vi "Main.vi"() -> ()   [LabVIEW 2016]
doc: "The myRIO Project template acquires acceleration data from the onboard accelerometer and displays the changes of acceleration values in a waveform chart."
uses:
  <vilib>/myRIO/Instrument Drivers/Onboard IO/PWM/typedefs/PWM Reference.ctl
  <vilib>/myRIO/Common/Instrument Driver Framework/Utilities/typedefs/myRIO Generic Hardware Reference.ctl
  <vilib>/myRIO/Common/Instrument Driver Framework/Utilities/typedefs/Hardware Version Enum.ctl
  <vilib>/myRIO/Common/Instrument Driver Framework/Utilities/typedefs/myRIO v1.0 Reference.ctl
  <vilib>/myRIO/Common/Instrument Driver Framework/Utilities/typedefs/Generic FPGA Reference.ctl
  <vilib>/myRIO/Common/Instrument Driver Framework/myRIO v1.0/PWM/typedefs/PWM Channels Enum.ctl
  <vilib>/myRIO/Instrument Drivers/Onboard IO/PWM/typedefs/PWM Configuration.ctl
  <vilib>/userdefined/High Color/nirio_resource_hc.ctl
  <vilib>/myRIO/Common/Instrument Driver Framework/myRIO v1.0/PWM/vis/myRIO v1.1 Open PWM.vi
  <vilib>/myRIO/Common/Instrument Driver Framework/Utilities/vis/Validate Channels.vi
  <vilib>/myRIO/Common/Instrument Driver Framework/myRIO v1.0/PWM/vis/myRIO v1.0 Reserve PWM.vi
  <vilib>/myRIO/Instrument Drivers/Onboard IO/PWM/vis/Set Duty Cycle and Frequency.vi
  <vilib>/myRIO/Common/Instrument Driver Framework/myRIO v1.0/PWM/vis/myRIO v1.0 Close PWM.vi
  <vilib>/myRIO/Common/Instrument Driver Framework/myRIO v1.0/UART/vis/myRIO v1.0 Close UART.vi
  <vilib>/myRIO/Common/Instrument Driver Framework/myRIO v1.0/PWM/vis/myRIO v1.0 Build MUX Configuration PWM.vi
  <vilib>/myRIO/Common/Instrument Driver Framework/myRIO v1.0/Resource Manager/vis/myRIO v1.0 Reserve Channel List.vi
  <vilib>/myRIO/Common/Instrument Driver Framework/myRIO v1.0/PWM/vis/myRIO v1.0 Unreserve PWM.vi
  <vilib>/myRIO/Common/Instrument Driver Framework/myRIO v1.0/Resource Manager/vis/myRIO v1.0 Create Configuration List.vi
  <vilib>/myRIO/Common/Instrument Driver Framework/myRIO v1.0/Resource Manager/vis/myRIO v1.0 Reserve Channel.vi
  <vilib>/myRIO/Common/Instrument Driver Framework/myRIO v1.0/Resource Manager/vis/myRIO v1.0 Unreserve Channel.vi
  <vilib>/myRIO/Common/Instrument Driver Framework/myRIO v1.0/Resource Manager/vis/myRIO v1.0 Unreserve Channel List.vi
  <vilib>/myRIO/Common/Instrument Driver Framework/myRIO v1.0/Resource Manager/vis/myRIO v1.0 Build Mutex Name.vi
  <vilib>/Utility/VariantDataType/GetNumericInfo.vi
  <vilib>/Utility/error.llb/Error Cluster From Error Code.vi
  <vilib>/myRIO/Common/Instrument Driver Framework/myRIO v1.0/myRIO v1.1 Open.vi
  <vilib>/myRIO/Common/Instrument Driver Framework/Utilities/vis/IO Manager.vi
  <vilib>/myRIO/Common/Instrument Driver Framework/Utilities/vis/Configuration Manager.vi
  <vilib>/myRIO/Common/Instrument Driver Framework/myRIO v1.0/Resource Manager/vis/myRIO v1.0 Configure IO.vi
  <vilib>/myRIO/Common/Instrument Driver Framework/myRIO v1.0/myRIO v1.0 Close.vi
  <vilib>/myRIO/Common/Instrument Driver Framework/myRIO v1.0/PWM/vis/myRIO v1.0 Write PWM.vi
  <vilib>/myRIO/Common/Instrument Driver Framework/myRIO v1.0/PWM/vis/myRIO v1.0 Shutdown PWM.vi
  <vilib>/myRIO/Common/Instrument Driver Framework/Utilities/vis/FPGA Ref Manager.vi
  <vilib>/myRIO/Common/Instrument Driver Framework/myRIO v1.0/myRIO v1.0 Reset FPGA.vi
  <vilib>/myRIO/Common/Instrument Driver Framework/myRIO v1.0/IRQ/vis/myRIO v1.0 IRQ Info FGV.vi
  <vilib>/myRIO/Common/Instrument Driver Framework/myRIO v1.0/IRQ/vis/myRIO v1.0 Timer IRQ Info FGV.vi
  <vilib>/myRIO/Common/Instrument Driver Framework/myRIO v1.0/IRQ/vis/myRIO v1.0 ISR Agent.vi
  <vilib>/myRIO/Instrument Drivers/Onboard IO/PWM/vis/myRIO PWM Open.xnode
  <vilib>/myRIO/Instrument Drivers/Utilities/Utilities.lvlib
  <vilib>/myRIO/Instrument Drivers/Onboard IO/PWM/PWM.lvlib
panel:
  in  "Blue Duty Cycle":dbl(slide)=10.0 scale=0.0..10.0
  in  "Green Duty Cycle":dbl(slide)=10.0 scale=0.0..10.0
  in  "Red Duty Cycle":dbl(slide)=1.0 scale=0.0..1.0
  in  "BlueChannel(2)":tag="A/PWM2"
  in  "GreenChannel(1)":tag="A/PWM1"
  in  "RedChannel(0)":tag="A/PWM0"
  out "error out":errorcluster
  in  "Stop":bool
  # "Overview: The myRIO Project template acquires acceleration data from the onboard accelerometer and displays the changes of acceleration values in a waveform chart.\nInstructions:\n1. Check the myRIO target IP address in the project and make sure the target IP address is correct. \n2. Run this VI."
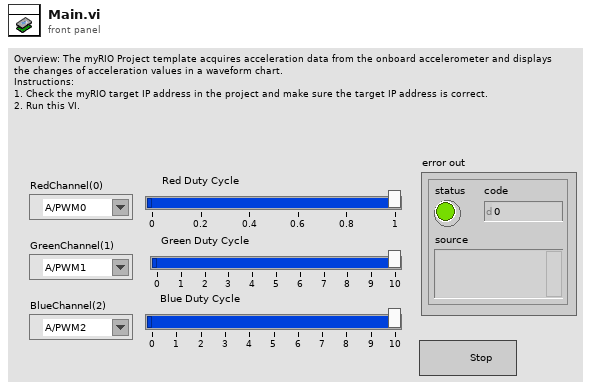
[diagram p1: front panel]
types:
  T1 = typedef "nirio_resource_hc.ctl" = tag
  T2 = typedef "Hardware Version Enum.ctl" = enum16{"Unknown", "myRIO-1900", "myRIO-1950", "roboRIO", "NI ELVIS RIO CM"}
  T3 = typedef "PWM.lvlib/PWM Reference.ctl" = cluster{"myRIO Reference":T4, "PWM Channels Enum":T7, "PWM Configuration":T8}
  T4 = typedef "myRIO Generic Hardware Reference.ctl" = cluster{"myRIO Model":T2, "myRIO Hardware Reference":T5}
  T5 = typedef "myRIO v1.0 Reference.ctl" = cluster{"Generic FPGA Reference":T6, "Allow multiple opens":bool}
  T6 = typedef "Generic FPGA Reference.ctl" = refnum<k20>
  T7 = typedef "PWM Channels Enum.ctl" = enum16{"Not Connected", "C/PWM0", "C/PWM1", "A/PWM0", "A/PWM1", "A/PWM2", "B/PWM0", "B/PWM1", "B/PWM2", "PWM/PWM0", "PWM/PWM1", "PWM/PWM2", "PWM/PWM3", "PWM/PWM4", "PWM/PWM5", "PWM/PWM6", "PWM/PWM7", "PWM/PWM8", "PWM/PWM9"}
  T8 = typedef "PWM.lvlib/PWM Configuration.ctl" = cluster{"Frequency":dbl, "Duty Cycle":dbl}
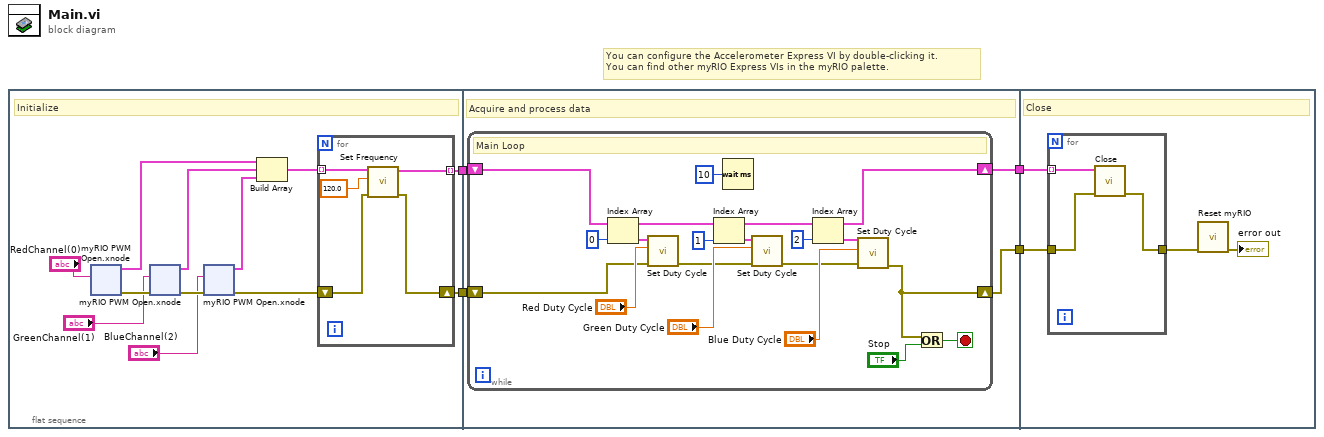
[diagram p0: block diagram]
diagram:
  # "You can configure the Accelerometer Express VI by double-clicking it.\nYou can find other myRIO Express VIs in the myRIO palette."
  n1 = flat-sequence {
    tunnel: [w10] -> w3
    tunnel: [w5] -> w2
    tunnel: [w73] -> w4
    tunnel: w3 -> [w72]
    tunnel: w2 -> [w71]
    tunnel: [w70] -> w1
    tunnel: w4 -> [w93]
    tunnel: w1 -> [w91]
    frame #0 {
      # "Initialize"
      n2 = xnode "myRIO PWM Open.xnode"("Channel Name"="RedChannel(0)") -> ("error out"=w15:errorcluster, "PWM Ref Out"=w9:T3)  [unwired: 2 in]
      n3 = xnode "myRIO PWM Open.xnode"("error in (no error)"=w15, "Channel Name"="GreenChannel(1)") -> ("error out"=w14:errorcluster, "PWM Ref Out"=w8:T3)  [unwired: 1 in]
      n4 = xnode "myRIO PWM Open.xnode"("error in (no error)"=w14, "Channel Name"="BlueChannel(2)") -> ("error out"=w11:errorcluster, "PWM Ref Out"=w7:T3)  [unwired: 1 in]
      n5 = Build Array(w9, w8, w7) -> (w6:T3[])
      n6 = for {
        tunnel: w6 -> [w21] mode=indexing
        tunnel: [w17] -> w5 mode=indexing
        shift-right: [w19] -> w10
        shift-left: w11 -> [w20]
        n7 = call <vilib>:"Set Frequency.vi"("error in (no error)"=w20, "Frequency [Hz]"=120.0, "PWM Ref In"=w21) -> ("error out"=w19:errorcluster, "PWM Ref Out"=w17:T3)  [unwired: 6 in]
      }
    }
    frame #1 {
      # "Acquire and process data"
      n8 = while {
        shift-right: [w74] -> w73
        shift-left: w72 -> [w77]
        shift-right: [w86] -> w70
        shift-left: w71 -> [w86]
        stop <- w89 stop-if-true
        # "Main Loop"
        n9 = Index Array(array=w86, index=0) -> (element=w87:T3)
        n10 = call <vilib>:"Set Duty Cycle.vi"("error in (no error)"=w77, "Duty Cycle"="Red Duty Cycle", "PWM Ref In"=w87) -> ("error out"=w76:errorcluster)  [unwired: 6 in, 1 out]
        n11 = Index Array(array=w86, index=1) -> (element=w82:T3)
        n12 = Wait (ms)(milliseconds to wait=u32 10) -> ()  [unwired: 1 out]
        n13 = call <vilib>:"Set Duty Cycle.vi"("error in (no error)"=w76, "Duty Cycle"="Green Duty Cycle", "PWM Ref In"=w82) -> ("error out"=w75:errorcluster)  [unwired: 6 in, 1 out]
        n14 = Index Array(array=w86, index=2) -> (element=w81:T3)
        n15 = call <vilib>:"Set Duty Cycle.vi"("error in (no error)"=w75, "Duty Cycle"="Blue Duty Cycle", "PWM Ref In"=w81) -> ("error out"=w74:errorcluster)  [unwired: 6 in, 1 out]
        n16 = Or(x=w74, y="Stop") -> (x .or. y?=w89:bool)
      }
    }
    frame #2 {
      # "Close"
      n17 = for {
        tunnel: w93 -> [w97]
        tunnel: [w96] -> w92
        tunnel: w91 -> [w95] mode=indexing
        n18 = call <vilib>:"Close.vi"("error in (no error)"=w97, "PWM Ref In"=w95) -> ("error out"=w96:errorcluster)  [unwired: 9 in]
      }
      n19 = call <vilib>:"Reset myRIO.vi"("error in (no error)"=w92) -> ("error out"=→"error out":errorcluster)  [unwired: 10 in]
    }
  }
